vi "_s_Extract_SN.vi"(8 "error in (no error)":errorcluster, 10 "Read String":string) -> (0 "error out":errorcluster, 1 "Reading":T1, 2 "Result":string)   [LabVIEW 2013]
panel:
  out "Command":string
  out "Param":string
  out "Process":string
  out "Node":string
  out "Lenght":string
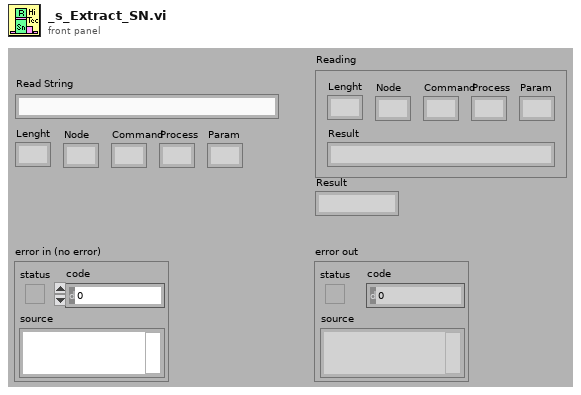
[diagram p1: front panel]
types:
  T1 = cluster{"Lenght":string, "Node":string, "Process":string, "Param":string, "Command":string, "Result":string}
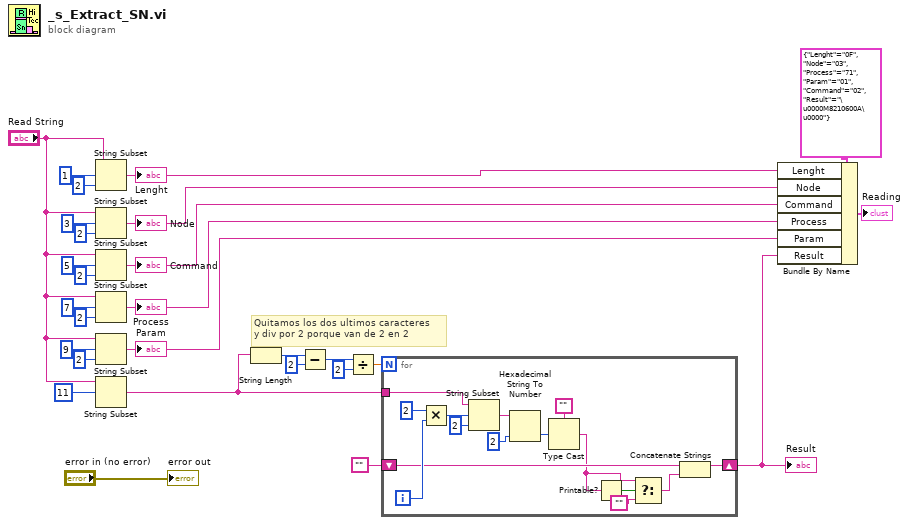
[diagram p0: block diagram]
diagram:
  # "Quitamos los dos ultimos caracteres\ny div por 2 porque van de 2 en 2"
  n1 = String Subset(string="Read String", offset (0)=1, length (rest)=2 ("length (rest)")) -> (substring=w9:string)
  "Lenght" <- w9
  n2 = String Subset(string="Read String", offset (0)=3, length (rest)=2 ("length (rest)")) -> (substring=w8:string)
  "Node" <- w8
  n3 = String Subset(string="Read String", offset (0)=5, length (rest)=2 ("length (rest)")) -> (substring=w7:string)
  "Command" <- w7
  n4 = String Subset(string="Read String", offset (0)=7, length (rest)=2 ("length (rest)")) -> (substring=w6:string)
  "Process" <- w6
  n5 = String Subset(string="Read String", offset (0)=9, length (rest)=2 ("length (rest)")) -> (substring=w5:string)
  "Param" <- w5
  n6 = String Subset(string="Read String", offset (0)=11) -> (substring=w1:string)  [unwired: 1 in]
  n7 = String Length(string=w1) -> (length=w28:i32)
  n8 = Subtract(x=w28, y=2) -> (x-y=w25:i32)
  n9 = Divide(x=w25, y=2) -> (x/y=w12:dbl)
  n10 = for {
    N: w12 -> [_]
    tunnel: w1 -> [w39]
    shift-right: [w35] -> w4
    shift-left: "" ("Empty String Constant") -> [w36]
    i -> [w41]
    n11 = Multiply(x=2 ("length (rest)"), y=w41) -> (x*y=w40:i32)
    n12 = String Subset(string=w39, offset (0)=w40, length (rest)=2 ("length (rest)")) -> (substring=w38:string)
    n13 = Hexadecimal String To Number(string=w38, default (0uL)=u8 2 ("length (rest)")) -> (number=w37:u8)  [unwired: 1 in, 1 out]
    n14 = Type Cast(type="" ("Empty String Constant"), x=w37) -> (*(type *) &x=w31:string)
    n15 = Printable?(1:w31) -> (0:w32:bool)
    n16 = Select(t=w31, s=w32, f="" ("Empty String Constant")) -> (s? t:f=w30:string)
    n17 = Concatenate Strings(w36, w30) -> (w35:string)
  }
  "Result" <- w4
  n18 = Bundle By Name(cluster=T1 {"Lenght"="0F", "Node"="03", "Process"="71", "Param"="01", "Command"="02", "Result"="\u0000M8210600A\u0000"} ("Reading"), "Lenght"=w9, "Node"=w8, "Command"=w7, "Process"=w6, "Param"=w5, "Result"=w4) -> (→"Reading":T1)
  "error out" <- "error in (no error)"
